vi "Fix Drift in File.vi"(7 "End field value":dbl, 8 "error in (no error)":errorcluster, 9 "channel name(s) in":string="Field", 10 "group name":string="Untitled", 11 "tdms file":refnum<k34>) -> (0 "error out":errorcluster, 1 "Min max":cluster{"Max":dbl, "Min":dbl}, 2 "Max field":dbl, 3 "tdms file out":refnum<k34>, 4 "channel name(s) out":string)   [LabVIEW 2016]
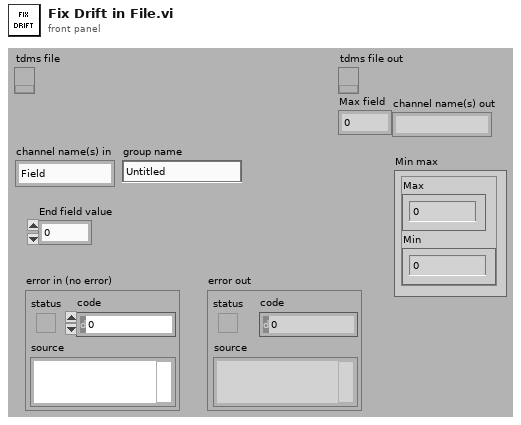
[diagram p1: front panel]
types:
  T1 = enum16{"open", "open or create", "create or replace", "create", "open (read-only)"}
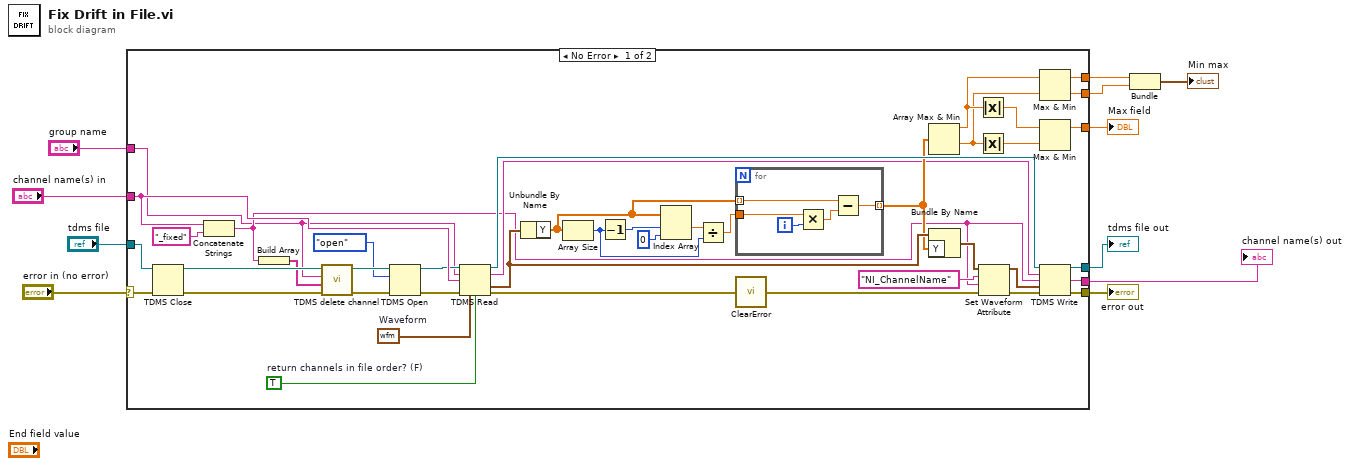
[diagram p0: block diagram]
diagram:
  n1 = case shown="No Error" "error in (no error)" {
    selector: "error in (no error)" -> [w27 w59]
    tunnel: [w47 w59] -> w11
    tunnel: [w31 _] -> w9
    tunnel: [w30 _] -> w8
    tunnel: "tdms file" -> [w17 _]
    tunnel: "group name" -> [w13 _]
    tunnel: "channel name(s) in" -> [w23 _]
    tunnel: [w15 _] -> w3
    tunnel: [w14 _] -> w2
    tunnel: [w12 _] -> w1
    frame No Error {
      w34 = TRUE  # return channels in file order? (F)
      w53 = waveform(dbl) {"t0"=timestamp(0 s since 1904-01-01), "dt"=1.0, "Y"=[]}  # Waveform
      n2 = TDMS Close(8:w27, 11:w17) -> (0:w25:errorcluster, 3:w26:path)
      n3 = Concatenate Strings(w23, "_fixed" ("string")) -> (w22:string)
      n4 = Build Array(w22) -> (w24:string[])
      n5 = call "TDMS delete channel.vi"("error in (no error)"=w25, "Channels"=w24, "group name"=w13, "file path"=w26) -> ("error out"=w19:errorcluster, "file path out"=w21:path)  [unwired: 5 in, 1 out]
      n6 = TDMS Open(8:w19, 10:T1."open" ("operation (0:open)"), 11:w21) -> (0:w18:errorcluster, 3:w16:refnum<k34>)  [unwired: 4 in]
      n7 = TDMS Read(0:w16, 5:w13, 7:w23, 11:w18, 12:w53, 13:w34) -> (4:w45:refnum<k34>, 6:w28:string, 10:w44:waveform(dbl), 15:w38:errorcluster)  [unwired: 2 in, 2 out]
      n8 = Unbundle By Name(w44) -> ("Y"=w41:dbl[])
      n9 = Array Size(array=w41) -> (size(s)=w42:i32)
      n10 = Decrement(x=w42) -> (x-1=w40:i32)
      n11 = Index Array(array=w41, index #1=w40, index #2=0 ("index")) -> (element #1=w39:dbl)  [unwired: 1 out]
      n12 = Divide(x=w39, y=w42) -> (x/y=w52:dbl)
      n13 = for {
        tunnel: w41 -> [w58] mode=indexing
        tunnel: w52 -> [w56]
        tunnel: [w54] -> w37 mode=indexing
        i -> [w57]
        n14 = Multiply(x=w56, y=w57) -> (x*y=w55:dbl)
        n15 = Subtract(x=w58, y=w55) -> (x-y=w54:dbl)
      }
      n16 = call <vilib>:"ClearError.vi"("error in (no error)"=w38) -> ("error out"=w43:errorcluster)
      n17 = Array Max & Min(array=w37) -> (max value=w33:dbl, min value=w32:dbl)  [unwired: 2 out]
      n18 = Bundle By Name(cluster=w44, "Y"=w37) -> (w50:waveform(dbl))
      n19 = Absolute Value(x=w33) -> (abs(x)=w36:dbl)
      n20 = Absolute Value(x=w32) -> (abs(x)=w35:dbl)
      n21 = Set Waveform Attribute(4:w43, 5:w22, 6:"NI_ChannelName" ("name"), 7:w50) -> (0:w48:errorcluster, 3:w46:waveform(dbl))  [unwired: 1 out]
      n22 = Max & Min(x=w33, y=w32) -> (max(x,y)=w31:dbl, min(x,y)=w30:dbl)
      n23 = Max & Min(x=w36, y=w35) -> (max(x,y)=w15:dbl)  [unwired: 1 out]
      n24 = TDMS Write(0:w45, 5:w28, 7:w22, 9:w46, 11:w48) -> (4:w14:refnum<k34>, 8:w12:string, 15:w47:errorcluster)  [unwired: 1 in, 1 out]
    }
    frame Error {
    }
  }
  "error out" <- w11
  "Max field" <- w3
  "tdms file out" <- w2
  "channel name(s) out" <- w1
  n25 = Bundle(w9, w8) -> (→"Min max":cluster{dbl, dbl})  [unwired: 1 in]
